vi "Get Element Info of Variant.vi"(8 "error in (no error)":errorcluster, 11 "Data Type":variant) -> (0 "error out":errorcluster, 1 "Array Element Size":i32, 2 "Array Size":i32, 3 "Total Size":i32, 4 "Cluster Info":T1[](array[typedef]), 5 "Array":bool)   [LabVIEW 2021, in "DataTypes_CIF_U.lvlib"]
uses:
  DataTypes_CIF_U.lvlib
  <vilib>/Utility/Data Type/NI_Data Type.lvlib
  Typedef/Errors.ctl
  <vilib>/Utility/Data Type/Type Definitions/Data Type.ctl
  Typedef/Cluster Info.ctl
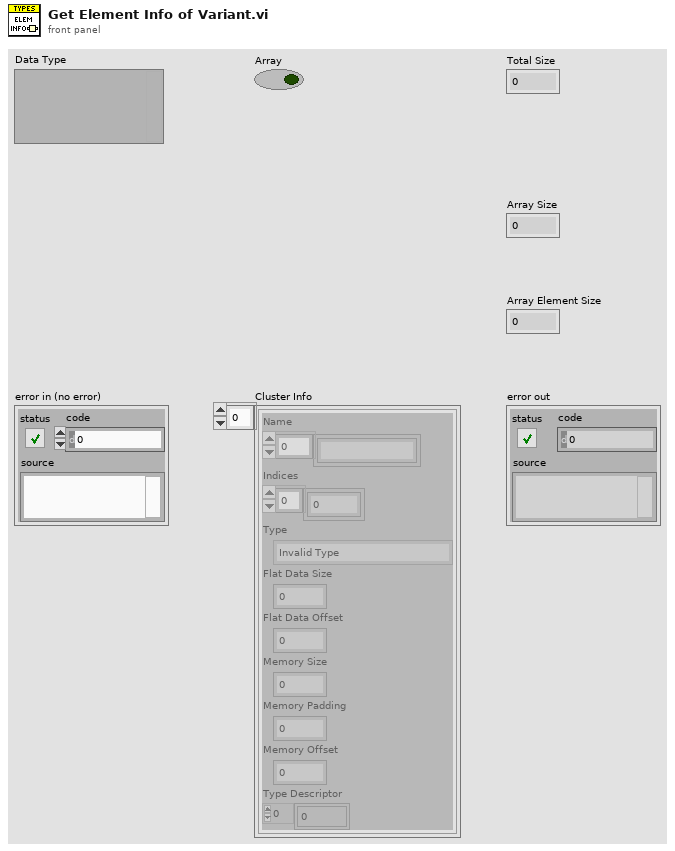
[diagram p1: front panel]
types:
  T1 = typedef "DataTypes_CIF_U.lvlib/Cluster Info.ctl" = cluster{"Name":string[], "Indices":i32[], "Type":T2, "Flat Data Size":u32, "Flat Data Offset":u32, "Memory Size":u32, "Memory Padding":u32, "Memory Offset":u32, "Type Descriptor":i16[]}
  T2 = typedef "NI_Data Type.lvlib/Data Type.ctl" = enum8{"Invalid Type", "Void", "I8", "I16", "I32", "I64", "U8", "U16", "U32", "U64", "Single Float", "Double Float", "Extended Float", "Single Complex", "Double Complex", "Extended Complex", "Enum U8", "Enum U16", "Enum U32", "Enum U64", "Single Float With Unit", "Double Float With Unit", "Extended Float With Unit", "Single Complex with Unit", "Double Complex with Unit", "Extended Complex with Unit", "Boolean", "String", "Path", "Picture", "Tag", "Array", "Cluster", "Variant", "LV Variant", "Waveform", "Timestamp", "Digital Waveform", "Digital Data", "ExpressData", "Refnum", "External Data", "VI", "Poly VI", "LabVIEW Class Instance", "Fixed Point", "Set Collection", "Map Collection"}
  T3 = typedef "DataTypes_CIF_U.lvlib/Errors.ctl" = enum16{"Too few bytes", "Unsupported Type", "Invalid GUID"}
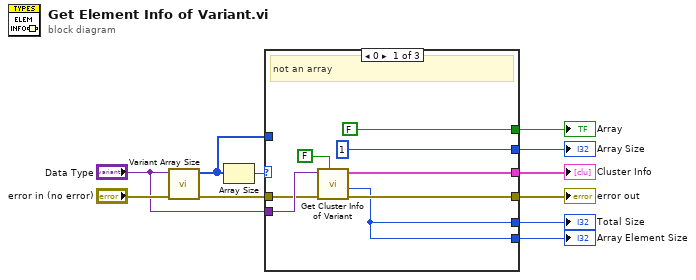
[diagram p0: block diagram]
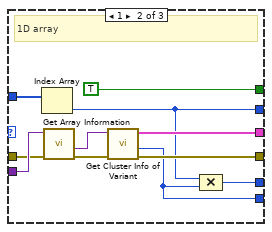
[diagram p2: hidden frame]
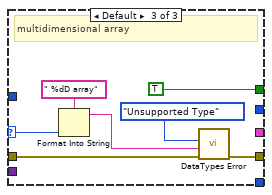
[diagram p3: hidden frame]
diagram:
  n1 = call "Variant Array Size.vi"("error in (no error)"="error in (no error)", "data"="Data Type") -> ("error out"=w9:errorcluster, "lengths"=w1:i32[])  [unwired: 7 in, 1 out]
  n2 = Array Size(array=w1) -> (size(s)=w10:i32)
  n3 = case shown="0" w10 {
    selector: w10 -> [_ _ w35]
    tunnel: w9 -> [w18 w20 w34]
    tunnel: "Data Type" -> [w19 w21 _]
    tunnel: [w17 w27 w32] -> w7
    tunnel: [w13 w24 _] -> w6
    tunnel: [w13 w25 _] -> w5
    tunnel: [w16 w23 _] -> w4
    tunnel: [1 ("array_size") w22 _] -> w3
    tunnel: [FALSE ("is_array?") TRUE ("is_array?") TRUE ("is_array?")] -> w2
    tunnel: w1 -> [_ w26 _]
    frame 0 {
      # "not an array"
      n4 = call "Get Cluster Info of Variant.vi"("Append Cluster Name"=FALSE, "error in (no error)"=w18, "Cluster Variant"=w19) -> ("error out"=w17:errorcluster, "mem_size"=w13:i32, "Cluster Info"=w16:T1[])  [unwired: 4 in, 2 out]
    }
    frame 1 {
      # "1D array"
      n5 = Index Array(array=w26) -> (element=w22:i32)  [unwired: 1 in]
      n6 = call <vilib>:"Get Array Information.vi"("error in (no error)"=w20, "variant"=w21) -> ("error out"=w28:errorcluster, "array element data type"=w29:variant)  [unwired: 6 in, 2 out]
      n7 = call "Get Cluster Info of Variant.vi"("error in (no error)"=w28, "Cluster Variant"=w29) -> ("error out"=w27:errorcluster, "mem_size"=w24:i32, "Cluster Info"=w23:T1[])  [unwired: 5 in, 2 out]
      n8 = Compound Arithmetic op=MULTIPLY(w22, w24) -> (w25:i32)
    }
    frame Default {
      # "multidimensional array"
      n9 = Format Into String(format string=" %dD array", w35) -> (resulting string=w31:string)  [unwired: 2 in, 1 out]
      n10 = call "DataTypes Error.vi"("error in (no error)"=w34, "String to Append"=w31, "Error"=Errors."Unsupported Type") -> ("error out"=w32:errorcluster)  [unwired: 8 in]
    }
  }
  "Total Size" <- w5
  "Array" <- w2
  "Array Element Size" <- w6
  "error out" <- w7
  "Cluster Info" <- w4
  "Array Size" <- w3
